vi "Outputs.vi"() -> ()   [LabVIEW 2017]
panel:
  in  "Vp":dbl
  in  "Vy":dbl
  in  "Vx":dbl
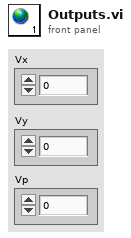
[diagram p1: front panel]
diagram:
